vi "Agilent DMM Read Null State.vi"(8 "error in (no error)":errorcluster, 11 "VISA Resource Name":refnum<visa-resource-name>) -> (0 "error out":errorcluster, 1 "Null Value":dbl, 2 "Calibrated?":bool, 3 "dup VISA Resource Name":refnum<visa-resource-name>)   [LabVIEW 2011]
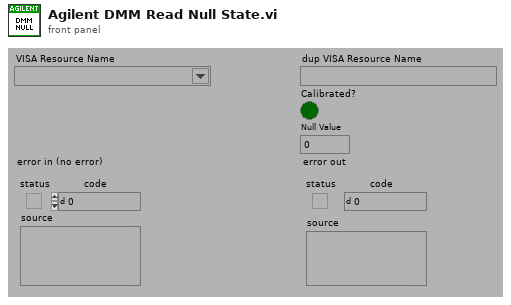
[diagram p1: front panel]
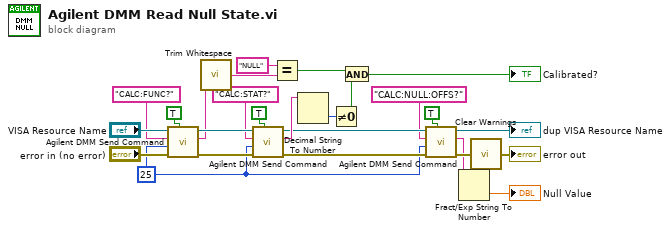
[diagram p0: block diagram]
diagram:
  w6 = u32 25 ("byte count")
  n1 = call "Agilent DMM Send Command.vi"("Read? (F)"=TRUE, "error in (no error)"="error in (no error)", "Byte Count"=w6, "Command"="CALC:FUNC?", "VISA Resource Name"="VISA Resource Name") -> ("error out"=w18:errorcluster, "Data Read"=w1:string, "dup VISA Resource Name"=w19:refnum<visa-resource-name>)  [unwired: 4 out]
  n2 = call <vilib>:"Trim Whitespace.vi"("string"=w1) -> ("trimmed string"=w2:string)  [unwired: 1 in]
  n3 = call "Agilent DMM Send Command.vi"("Read? (F)"=TRUE, "error in (no error)"=w18, "Byte Count"=w6, "Command"="CALC:STAT?", "VISA Resource Name"=w19) -> ("error out"=w9:errorcluster, "Data Read"=w16:string, "dup VISA Resource Name"=w10:refnum<visa-resource-name>)  [unwired: 4 out]
  n4 = Equal?(x="NULL", y=w2) -> (x = y?=w13:bool)
  n5 = Decimal String To Number(string=w16) -> (number=w15:i32)  [unwired: 3 out]
  n6 = Not Equal To 0?(x=w15) -> (x != 0?=w14:bool)
  n7 = And(x=w13, y=w14) -> (x .and. y?=→"Calibrated?":bool)
  n8 = call "Agilent DMM Send Command.vi"("Read? (F)"=TRUE, "error in (no error)"=w9, "Byte Count"=w6, "Command"="CALC:NULL:OFFS?", "VISA Resource Name"=w10) -> ("error out"=w8:errorcluster, "Data Read"=w4:string, "dup VISA Resource Name"=→"dup VISA Resource Name":refnum<visa-resource-name>)  [unwired: 4 out]
  n9 = Fract/Exp String To Number(string=w4) -> (number=→"Null Value":dbl)  [unwired: 4 out]
  n10 = call "Clear Warnings.vi"("error in (no error)"=w8) -> ("error out"=→"error out":errorcluster)
